vi "Control Experiment Class to JSON.vi"(8 "error in (no error)":errorcluster, 11 "Control Experiment in":refnum<class "Control Experiment.lvclass">) -> (0 "error out":errorcluster, 2 "<JSON>":string, 3 "Control Experiment out":refnum<class "Control Experiment.lvclass">)   [LabVIEW 2019, in "Control Experiment.lvclass"]
uses:
  Control Experiment.lvclass
  04488a64-0300-4bba-8508-2a660ee34928.vi
  Typedefs/Instrument Types--enum.ctl
  Typedefs/Wiring Description--cluster.ctl
  Typedefs/Experiment Description--cluster.ctl
  Typedefs/Control Experiment FGV.JSON--cluster.ctl
  Typedefs/Instruments--cluster.ctl
  <vilib>/Utility/Data Type/NI_Data Type.lvlib
  Attributes/Instrument Attributes.lvlib
  <userlib>/LevyLab/Instrument Framework/Instrument/Instrument.lvclass
  C:/Program Files (x86)/National Instruments/LabVIEW 2019/vi.lib/JKI/JKI SMO/SMO/SMO.lvclass
  <userlib>/LevyLab/Instrument Framework/Instrument Types/Lockin/Instrument.LockinAPI.lvclass
  <userlib>/LevyLab/Instrument Framework/Instrument Types/Amplifier/Instrument.Amplifier.lvclass
  <userlib>/LevyLab/Instrument Framework/Instrument Types/Cryostat/Instrument.Cryostat.lvclass
  <userlib>/LevyLab/Instrument Framework/Instrument Types/CBridge/Instrument.CBridge.lvclass
  <userlib>/LevyLab/Instrument Framework/Instrument Types/Delay Line/Instrument.DelayLine.lvclass
  <userlib>/LevyLab/Instrument Framework/Instrument Types/Strain/Instrument.Strain.lvclass
  <userlib>/LevyLab/Instrument Framework/Instrument Types/VNA/Instrument.VNA.lvclass
  <userlib>/LevyLab/Instrument Framework/Instrument Types/VSource/Instrument.VSource.lvclass
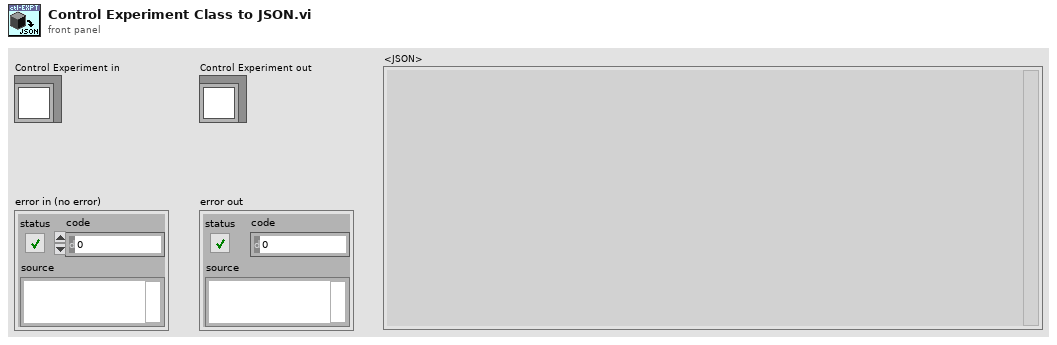
[diagram p1: front panel]
types:
  T1 = typedef "Control Experiment.lvclass/Control Experiment FGV.JSON--cluster.ctl" = cluster{"json":string, "Experiment":T2, "Wiring Configuration":T5}
  T2 = typedef "Control Experiment.lvclass/Experiment Description--cluster.ctl" = cluster{"User":string, "Device":string, "Device Path":path, "Device Description":string, "Experiment Path":path, "Experiment Description":string, "Instrument":string, "Instruments":T3[], "Sweep":cluster{"key":string, "value":variant}[]}
  T3 = typedef "Control Experiment.lvclass/Instruments--cluster.ctl" = cluster{"class path":path, "Address":string, "Type":T4}
  T4 = typedef "Control Experiment.lvclass/Instrument Types--enum.ctl" = enum16{"DAQ", "Amplifier", "Temperature", "Magnet", "Rotator", "Level", "Capacitance", "Delay Line", "Strain Cell", "VNA", "Source"}
  T5 = typedef "Control Experiment.lvclass/Wiring Description--cluster.ctl" = cluster{"Lockin Ch":i32[], "KH":cluster{"Electrodes":string[], "Labels":string[]}, "not KH":cluster{"Electrodes":string[], "Labels":string[]}}
  T6 = typedef "Control Experiment.lvclass/Instrument Classes--cluster.ctl" = cluster{"DAQ":refnum<class "Instrument.LockinAPI.lvclass">, "Amplifier":refnum<class "Instrument.Amplifier.lvclass">, "Temperature":refnum<class "Instrument.Cryostat.lvclass">, "Magnet":refnum<class "Instrument.Cryostat.lvclass">, "Rotator":refnum<class "Instrument.Cryostat.lvclass">, "Level":refnum<class "Instrument.Cryostat.lvclass">, "Capacitance":refnum<class "Instrument.CBridge.lvclass">, "Delay Line":refnum<class "Instrument.DelayLine.lvclass">, "Strain Cell":refnum<class "Instrument.Strain.lvclass">, "VNA":refnum<class "Instrument.VNA.lvclass">, "Source":refnum<class "Instrument.VSource.lvclass">}
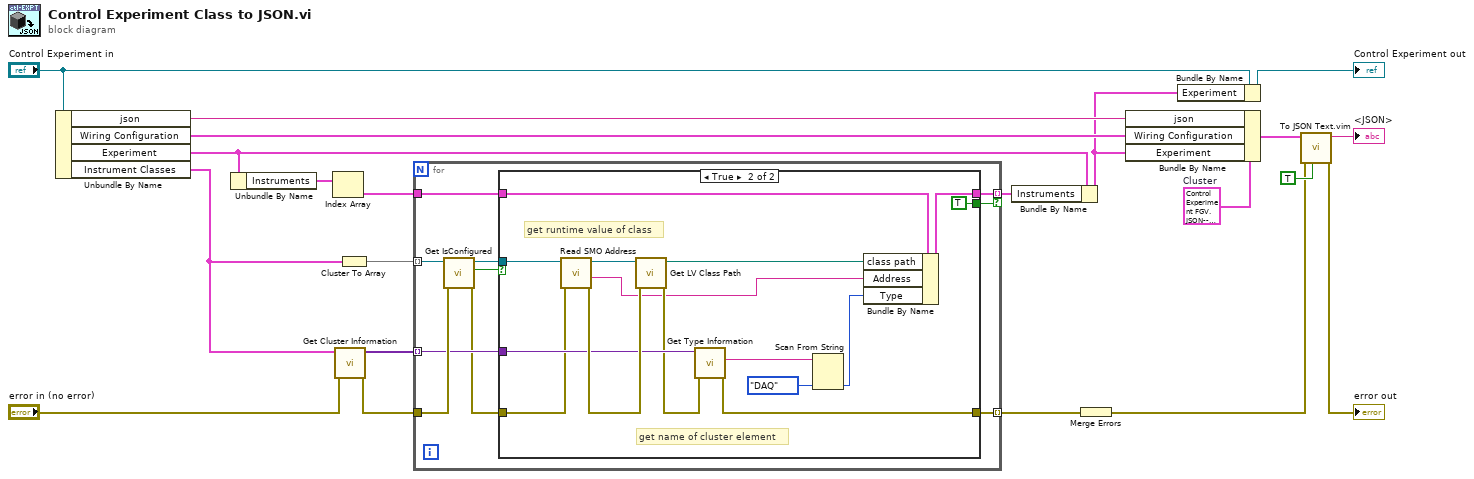
[diagram p0: block diagram]
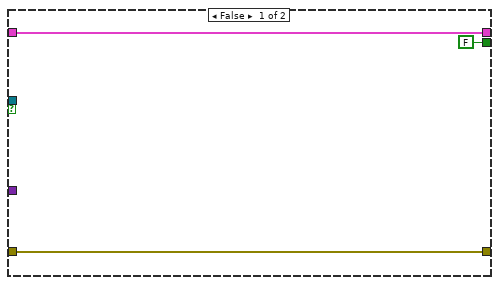
[diagram p2: hidden frame]
diagram:
  w8 = T1 {"json"="", "Experiment"={"User"="", "Device"="", "Device Path"=path "", "Device Description"="", "Experiment Path"=path "", "Experiment Description"="", "Instrument"="", "Instruments"=[], "Sweep"=[]}, "Wiring Configuration"={"Lockin Ch"=[], "KH"={"Electrodes"=[], "Labels"=[]}, "not KH"={"Electrodes"=[], "Labels"=[]}}}  # Cluster
  n1 = Unbundle By Name("Control Experiment in") -> ("json"=w9:string, "Wiring Configuration"=w14:T5, "Experiment"=w16:T2, "Instrument Classes"=w5:T6)
  n2 = Unbundle By Name(w16) -> ("Instruments"=w17:T3[])
  n3 = Index Array(array=w17) -> (element=w18:T3)  [unwired: 1 in]
  n4 = call <vilib>:"Get Cluster Information.vi"("error in (no error)"="error in (no error)", "variant"=w5) -> ("error out"=w1:errorcluster, "cluster elements"=w4:variant[])  [unwired: 8 in]
  n5 = Cluster To Array(cluster=w5) -> (array=w3:refnum<class "Instrument.lvclass">[])
  n6 = for {
    tunnel: w3 -> [w28] mode=indexing
    tunnel: [w31] -> w15 mode=indexing if=w22
    tunnel: w18 -> [w30]
    tunnel: w1 -> [w27]
    tunnel: [w25] -> w20 mode=indexing
    tunnel: w4 -> [w26] mode=indexing
    n7 = call "Get IsConfigured.vi"("error in (no error)"=w27, "SMO"=w28) -> ("error out"=w24:errorcluster, "IsConfigured?"=w23:bool, "SMO out"=w29:refnum<class "Instrument.lvclass">)  [unwired: 7 in]
    n8 = case shown="True" w23 {
      tunnel: [w34 w47] -> w31
      tunnel: w30 -> [w34 w46]
      tunnel: w29 -> [_ w41]
      tunnel: w26 -> [_ w40]
      tunnel: [w32 w38] -> w25
      tunnel: w24 -> [w32 w37]
      tunnel: [FALSE TRUE] -> w22
      frame False {
      }
      frame True {
        # "get runtime value of class"
        # "get name of cluster element"
        n9 = call <userlib>:"Read SMO Address.vi"("error in (no error)"=w37, "Instrument in"=w41) -> ("error out"=w48:errorcluster, "URI"=w35:string, "Instrument out"=w49:refnum<class "Instrument.lvclass">)  [unwired: 6 in, 1 out]
        n10 = call <vilib>:"Get LV Class Path.vi"("error in (no error)"=w48, "object"=w49) -> ("error out"=w39:errorcluster, "class path"=w45:path)  [unwired: 8 in]
        n11 = call <vilib>:"Get Type Information.vi"("error in (no error)"=w39, "variant"=w40) -> ("error out"=w38:errorcluster, "name"=w42:string)  [unwired: 5 in, 3 out]
        n12 = Scan From String(input string=w42, default 1=Instrument_Types--enum."DAQ" ("Type")) -> (output 1=w43:T4)  [unwired: 3 in, 3 out]
        n13 = Bundle By Name(cluster=w46, "class path"=w45, "Address"=w35, "Type"=w43) -> (w47:T3)
      }
    }
  }
  n14 = Bundle By Name(cluster=w16, "Instruments"=w15) -> (w7:T2)
  n15 = Merge Errors(w20) -> (w13:errorcluster)
  n16 = Bundle By Name(cluster=w8, "json"=w9, "Wiring Configuration"=w14, "Experiment"=w7) -> (w6:T1)
  n17 = Bundle By Name(cluster="Control Experiment in", "Experiment"=w7) -> (→"Control Experiment out":refnum<class "Control Experiment.lvclass">)
  n18 = call "To JSON Text.vim"("Pretty Print?"=TRUE, "error in (no error)"=w13, "Anything"=w6) -> ("error out"=→"error out":errorcluster, "<JSON>"=→"<JSON>":string)  [unwired: 7 in]
